vi "Ex2CamerasSameGraph.vi"() -> ()   [LabVIEW 2010]
panel:
  out "Camera 2":sgl[](graph)
  out "Camera 1":sgl[](graph)
  in  "stop 2":bool
  in  "stop":bool
  in  "Exposure Camera 2":dbl=0.5 format="%.2f"
  in  "Exposure Camera 1":dbl=0.5 format="%.2f"
  out "error out":errorcluster
  in  "error in (no error)":errorcluster
  # "Ex2CamerasSameGraph:\nThis example runs two cameras in focus mode.\nSets them up for center strip and displays as graph.\nRemember to setup two cameras in the pvcam.ini\nfile."
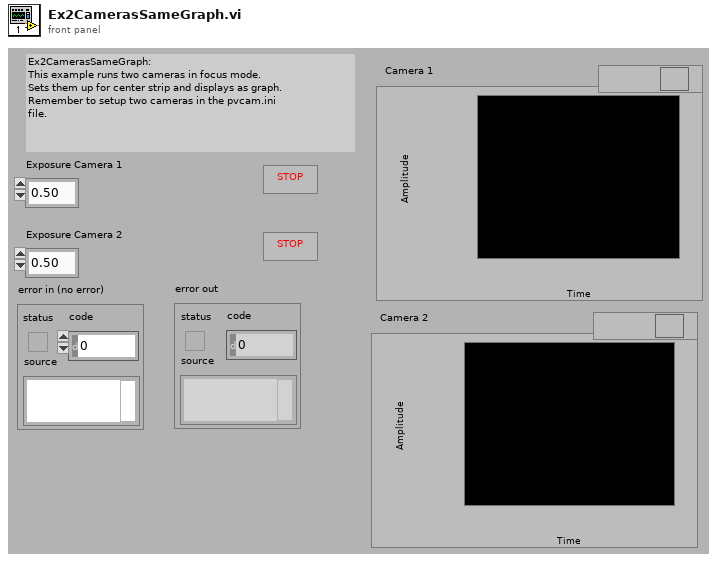
[diagram p1: front panel]
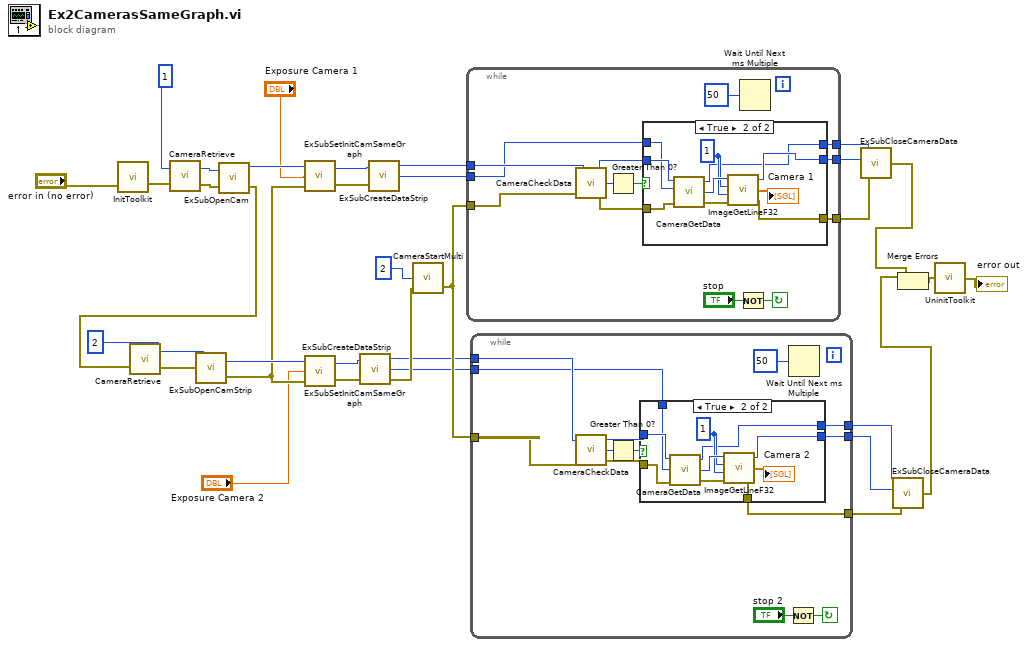
[diagram p0: block diagram]
diagram:
  n1 = call <userlib>:"InitToolkit.vi"("error in"="error in (no error)") -> ("error out"=w27:errorcluster)
  n2 = call <userlib>:"CameraRetrieve.vi"("error in"=w27, "Camera Index"=1) -> ("error out"=w29:errorcluster, "Device ID"=w28:u32)
  n3 = call "ExSubOpenCam.vi"("error in (no error)"=w29, "Camera Device ID"=w28) -> ("error out"=w23:errorcluster, "Camera Handle"=w34:u32)
  n4 = call <userlib>:"CameraRetrieve.vi"("error in"=w23, "Camera Index"=2) -> ("error out"=w24:errorcluster, "Device ID"=w25:u32)
  n5 = call "ExSubOpenCamStrip.vi"("error in (no error)"=w24, "Camera Device ID"=w25) -> ("error out"=w30:errorcluster, "Camera Handle"=w33:u32)
  n6 = call "ExSubSetInitCamSameGraph.vi"("error in (no error)"=w30, "Exposure"="Exposure Camera 1", "Camera Handle"=w34) -> ("error out"=w17:errorcluster, "Camera Handle 2"=w11:u32)
  n7 = call "ExSubSetInitCamSameGraph.vi"("error in (no error)"=w30, "Exposure"="Exposure Camera 2", "Camera Handle"=w33) -> ("error out"=w16:errorcluster, "Camera Handle 2"=w14:u32)
  n8 = call "ExSubCreateDataStrip.vi"("Camera Handle"=w14, "error in (no error)"=w16) -> ("Camera Handle"=w13:u32, "Data/Image Handle"=w12:u32, "error out"=w15:errorcluster)
  n9 = call "ExSubCreateDataStrip.vi"("Camera Handle"=w11, "error in (no error)"=w17) -> ("Camera Handle"=w10:u32, "Data/Image Handle"=w9:u32)  [unwired: 1 out]
  n10 = call "CameraStartMulti.vi"("error in (no error)"=w15, "Number Of Cameras"=2) -> ("error out"=w20:errorcluster)  [unwired: 1 in, 1 out]
  n11 = while {
    tunnel: w20 -> [w41]
    tunnel: [w45] -> w5
    tunnel: w10 -> [w39]
    tunnel: w9 -> [w38]
    tunnel: [w37] -> w4
    tunnel: [w36] -> w1
    stop <- w46 continue-if-true
    n12 = call <userlib>:"CameraCheckData.vi"("Camera Handle"=w39, "error in"=w41) -> ("Camera Handle"=w40:u32, "Number Of Frames Available"=w44:i32, "error out"=w42:errorcluster)
    n13 = Greater Than 0?(x=w44) -> (x > 0?=w43:bool)
    n14 = case shown="True" w43 {
      tunnel: [w51 w57] -> w45
      tunnel: w42 -> [w51 w56]
      tunnel: w40 -> [w50 w55]
      tunnel: w38 -> [w49 w54]
      tunnel: [w49 w53] -> w37
      tunnel: [w50 w52] -> w36
      frame False {
      }
      frame True {
        w58 = 1
        n15 = call <userlib>:"CameraGetData.vi"("error in"=w56, "Data Handle"=w54, "Camera Handle"=w55) -> ("error out"=w61:errorcluster, "Data Handle"=w59:u32, "Camera Handle"=w52:u32)
        n16 = call <userlib>:"ImageGetLineF32.vi"("error in"=w61, "Z Position"=w58, "Y Position"=w58, "Data Handle"=w59) -> ("error out"=w57:errorcluster, "Array F32"=→"Camera 1":sgl[], "Data Handle"=w53:u32)
      }
    }
    n17 = Not(x="stop") -> (.not. x?=w46:bool)
    n18 = Wait Until Next ms Multiple(millisecond multiple=u32 50) -> ()  [unwired: 1 out]
  }
  n19 = while {
    tunnel: w20 -> [w66]
    tunnel: [w71] -> w8
    tunnel: w13 -> [w65]
    tunnel: w12 -> [w64]
    tunnel: [w63] -> w3
    tunnel: [w62] -> w2
    stop <- w72 continue-if-true
    n20 = call <userlib>:"CameraCheckData.vi"("Camera Handle"=w65, "error in"=w66) -> ("Camera Handle"=w67:u32, "Number Of Frames Available"=w70:i32, "error out"=w68:errorcluster)
    n21 = Greater Than 0?(x=w70) -> (x > 0?=w69:bool)
    n22 = case shown="True" w69 {
      tunnel: [w77 w83] -> w71
      tunnel: w68 -> [w77 w82]
      tunnel: w67 -> [w76 w81]
      tunnel: w64 -> [w75 w80]
      tunnel: [w75 w79] -> w63
      tunnel: [w76 w78] -> w62
      frame False {
      }
      frame True {
        w85 = 1
        n23 = call <userlib>:"CameraGetData.vi"("error in"=w82, "Data Handle"=w80, "Camera Handle"=w81) -> ("error out"=w87:errorcluster, "Data Handle"=w86:u32, "Camera Handle"=w78:u32)
        n24 = call <userlib>:"ImageGetLineF32.vi"("error in"=w87, "Z Position"=w85, "Y Position"=w85, "Data Handle"=w86) -> ("error out"=w83:errorcluster, "Array F32"=→"Camera 2":sgl[], "Data Handle"=w79:u32)
      }
    }
    n25 = Not(x="stop 2") -> (.not. x?=w72:bool)
    n26 = Wait Until Next ms Multiple(millisecond multiple=u32 50) -> ()  [unwired: 1 out]
  }
  n27 = call "ExSubCloseCameraData.vi"("error in (no error)"=w5, "Image Handle"=w4, "Camera Handle"=w1) -> ("error out"=w6:errorcluster)
  n28 = call "ExSubCloseCameraData.vi"("error in (no error)"=w8, "Image Handle"=w3, "Camera Handle"=w2) -> ("error out"=w7:errorcluster)
  n29 = Merge Errors(w6, w7) -> (w32:errorcluster)
  n30 = call <userlib>:"UninitToolkit.vi"("error in"=w32) -> ("error out"=→"error out":errorcluster)
